vi "Gen_Random_Sine.vi"(11 "Sampling Info":T1={"Fs"=10000.0, "#s"=2000.0}) -> (3 "data":sgl[](graph))   [LabVIEW 2020]
uses:
  <vilib>/measure/NI_MABase.lvlib
  Controls/Sampling_Info.ctl
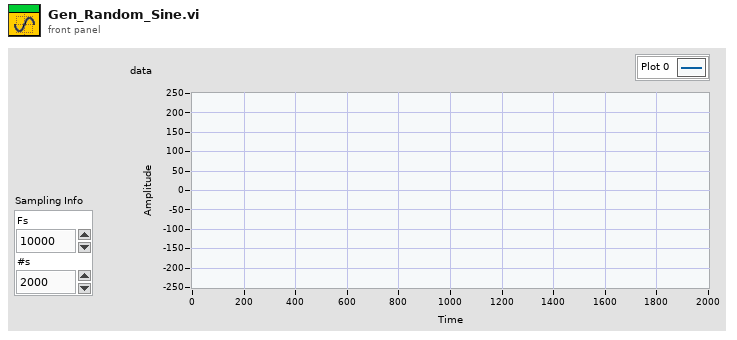
[diagram p1: front panel]
types:
  T1 = typedef "Sampling_Info.ctl" = cluster{"Fs":dbl, "#s":dbl}
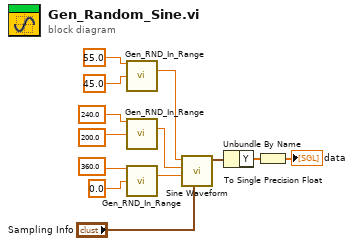
[diagram p0: block diagram]
diagram:
  n1 = call "Gen_RND_In_Range.vi"("Upper Bound"=55.0 ("frequency"), "Lower Bound"=45.0 ("Variation%")) -> ("RND_In_Range"=w9:dbl)  [unwired: 13 in]
  n2 = call "Gen_RND_In_Range.vi"("Upper Bound"=240.0 ("amplitude"), "Lower Bound"=200.0 ("variation")) -> ("RND_In_Range"=w8:dbl)  [unwired: 13 in]
  n3 = call "Gen_RND_In_Range.vi"("Upper Bound"=360.0 ("phase(digree)"), "Lower Bound"=0.0 ("Range")) -> ("RND_In_Range"=w5:dbl)  [unwired: 13 in]
  n4 = call <vilib>:"Sine Waveform.vi"("sampling info"="Sampling Info", "phase"=w5, "amplitude"=w8, "frequency"=w9) -> ("signal out"=w13:waveform(dbl))  [unwired: 6 in, 1 out]
  n5 = Unbundle By Name(w13) -> ("Y"=w12:dbl[])
  n6 = To Single Precision Float(number=w12) -> (single precision float=→"data":sgl[])
